vi "LaunchProcess.vi"(11 "SMO Reference":refnum<class "SMO.lvclass">) -> ()   [LabVIEW 2019, in "SMO.lvclass"]
doc: "Launches the Process VIs.\n\n---------------------------------------------------------------\nJKI State Machine Objects™\nhttp://jki.net/state-machine-objects/\nCopyright (C) 2005-2015, JKI <info@jki.net>\nALL RIGHTS RESERVEDJKI State Machine Objects (SMO) 1.3.0.56\nJKI - JKI\nCopyright (c) 2017, JKI"
uses:
  SMO.lvclass
panel:
  # "For instructions on how to use the JKI State Machine Objects, examples and video tutorials, visit:\nhttp://jki.net/state-machine-objects/\n\nJKI State Machine Objects™\nhttp://jki.net/state-machine-objects/\nCopyright (C) 2005-2015, JKI <info@jki.net>\nALL RIGHTS RESERVED"
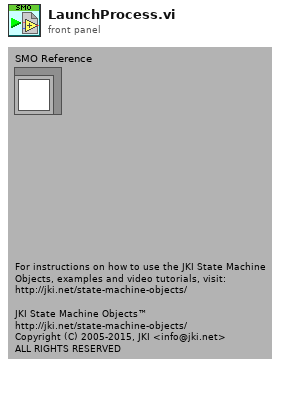
[diagram p1: front panel]
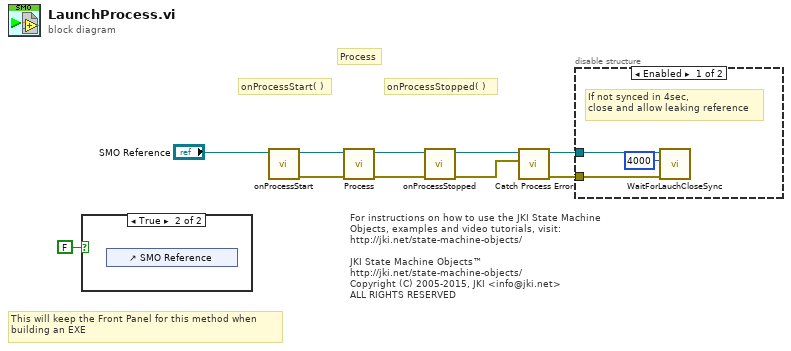
[diagram p0: block diagram]
diagram:
  # "Process"
  # "onProcessStart( )"
  # "onProcessStopped( )"
  # "This will keep the Front Panel for this method when\nbuilding an EXE"
  # "For instructions on how to use the JKI State Machine Objects, examples and video tutorials, visit:\nhttp://jki.net/state-machine-objects/\n\nJKI State Machine Objects™\nhttp://jki.net/state-machine-objects/\nCopyright (C) 2005-2015, JKI <info@jki.net>\nALL RIGHTS RESERVED"
  n1 = case shown="True" FALSE {
    frame False {
    }
    frame True {
      n2 = control-ref of="SMO Reference"() -> ()  [unwired: 1 out]
    }
  }
  n3 = call-dynamic "onProcessStart.vi"("SMO"="SMO Reference") -> ("error out"=w3:errorcluster, "SMO out"=w4:refnum<class "SMO.lvclass">)  [unwired: 9 in]
  n4 = call-dynamic "Process.vi"("error in"=w3, "SMO"=w4) -> ("error out"=w2:errorcluster, "SMO out"=w9:refnum<class "SMO.lvclass">)  [unwired: 8 in]
  n5 = call-dynamic "onProcessStopped.vi"("error in (no error)"=w2, "SMO"=w9) -> ("error out"=w1:errorcluster, "SMO out"=w8:refnum<class "SMO.lvclass">)  [unwired: 8 in]
  n6 = call "Catch Process Error.vi"("Process Error"=w1, "SMO"=w8) -> ("error out"=w6:errorcluster, "SMO out"=w7:refnum<class "SMO.lvclass">)  [unwired: 8 in]
  n7 = disable-structure shown="Enabled" {
    disable-tunnel: w7 -> [w13 _]
    disable-tunnel: w6 -> [w11 _]
    frame Enabled {
      # "If not synced in 4sec, \nclose and allow leaking reference"
      n8 = call "WaitForLauchCloseSync.vi"("error in (no error)"=w11, "timeout in ms (-1)"=4000, "SMO"=w13) -> ()  [unwired: 7 in, 2 out]
    }
    frame Disabled {
    }
  }
